vi "VFH, PID Test.vi"() -> ()   [LabVIEW 2016]
uses:
  <vilib>/Platform/TimedLoop/XDataNode/timing_clust.ctl
  <vilib>/Platform/TimedLoop/XDataNode/nitl_modes.ctl
  <vilib>/Platform/TimedLoop/XDataNode/wakeup.ctl
  <vilib>/Utility/AngleManip/Degrees to Radians (Scalar DBL).vi
  <vilib>/addons/control/pid/pid.llb/PID (DBL).vi
  <vilib>/addons/control/pid/pid.llb/PID Lead-Lag (DBL).vi
  <vilib>/Platform/TimedLoop/XDataNode/XDataNode.xnode
  <vilib>/express/express arith-compare/Formula/XNode/ExpressFormulaBlockNode.xnode
  <vilib>/Platform/TimedLoop/XDataNode/XDNodeRunTimeDep.lvlib
  <vilib>/addons/control/pid/NI_PID_pid.lvlib
  <vilib>/Utility/AngleManip/NI_AngleManipulation.lvlib
panel:
  in  "VFH ON/OFF":dbl
  out "Lidar_array":dbl[][](array[numeric])
  out "Encoder Speed_Filtered":dbl format="%#.8g"
  out "IMU Yaw_Filtered":dbl format="%#.8g"
  in  "Q":dbl[][](array[numeric])=[[0.001, 0.0], [0.0, 0.001]]
  in  "R":dbl[][](array[numeric])=[[1e-05, 0.0], [0.0, 1e-05]]
  out "Checksum":bool
  out "Valid":bool
  out "Speed_EKF":dbl
  out "GPS_Speed":dbl
  out "GPS_Heading angle":dbl
  out "Heading_EKF":dbl
  out "GPS_Longitude":dbl
  out "GPS_Latitude":dbl
  out "x_EKF":dbl
  out "y_EKF":dbl
  out "결과":dbl
  out "입력된 속도(protocol)":dbl
  out "Encoder Speed Filtered (m/s)":dbl
  in  "Platform_SPEED(테스트용)":u16
  in  "Lidar shift (m)":dbl=0.48
  in  "Vision shift (m)":dbl=0.87
  out "LIDAR & VISION DATA":cluster{dbl[], dbl[]}(graph)
  in  "Target angle":dbl
  out "Outer Threshold":dbl
  in  "Inner Threshold":dbl=1.5 format="%#_13g"
  in  "거리값 2":dbl
  out "현재 방향각":dbl
  out "Inner Threshold":dbl
  out "입력된 속도 (protocol)":u16
  in  "min speed (protocol)":dbl=35.0 format="%#_13g"
  in  "Global Stop":bool
  in  "Outer Threshold":dbl=0.68
  out "VFH error":bool
  out "PID 입력 브레이크":dbl
  in  "PID gains":T1={"proportional gain (Kc)"=1.0, "integral time (Ti, min)"=0.01, "derivative time (Td, min)"=0.0} caption="PID 게인" {"derivative time (Td, min)" format="%#.6g"; "integral time (Ti, min)" format="%#.6g"; "proportional gain (Kc)" format="%#.6g"}
  out "PV Setpoint Output":cluster{"initial PV":dbl, "setpoint":dbl}(graph)={"initial PV"=0.18693112703744846, "setpoint"=0.0}
  in  "PID 제동거리":dbl=0.5 format="%#_13g"
  in  "max speed (protocol)":dbl=50.0 format="%#_13g"
  in  "obstacle clearance distance":dbl=0.68
  out "mask":bool[](array[boolean])
  out "histogram":dbl[](array[numeric])
  out "Distance":dbl[](array[numeric])
  out "Angle":dbl[](array[numeric])
  in  "출력 클러스터 2":T2
  in  "탭 컨트롤":T3(tab)
  out "Vision Lane":dbl[][](array[numeric])
  out "Lidar 오브젝트화":dbl[][](array[numeric])
  out "Platform Data":i64[](array[numeric])
  out "IMU_Roll":dbl
  out "IMU_Pitch":dbl
  out "IMU_Acceleration":dbl
  out "Total Distance":dbl
  out "Encoder Speed":dbl
  out "IMU_Yaw":dbl
  out "ALIVE":u16
  in  "GEAR":u16(ring) items=["Forward Drive", "Neutral", "Backward Drive"]
  in  "A or M":bool=TRUE
  in  "Platform_E-STOP":bool
  in  "Lidar 오브젝트화 제한 거리(mm)":dbl=200.0
  in  "Lidar 필터 최대거리 (mm)":dbl=25000.0
  in  "Lidar 필터 최소거리 (mm)":dbl=50.0
  in  "GPS port num":refnum<visa-resource-name>="COM9"
  in  "IMU port num":refnum<visa-resource-name>="COM4"
  in  "LIDAR Address":string="192.168.0.204"
  in  "LIDAR port num":u16=2111
  in  "Platform port num":refnum<visa-resource-name>="COM6"
  out "End Loop":bool=TRUE
  # "GPS Data"
  # "IMU, Encoder Data"
  # "KF Data"
  # "EKF Data"
  # "VISION Lane"
  # "LIDAR Obstacle"
  # "Platform Data"
  # "Port Setting"
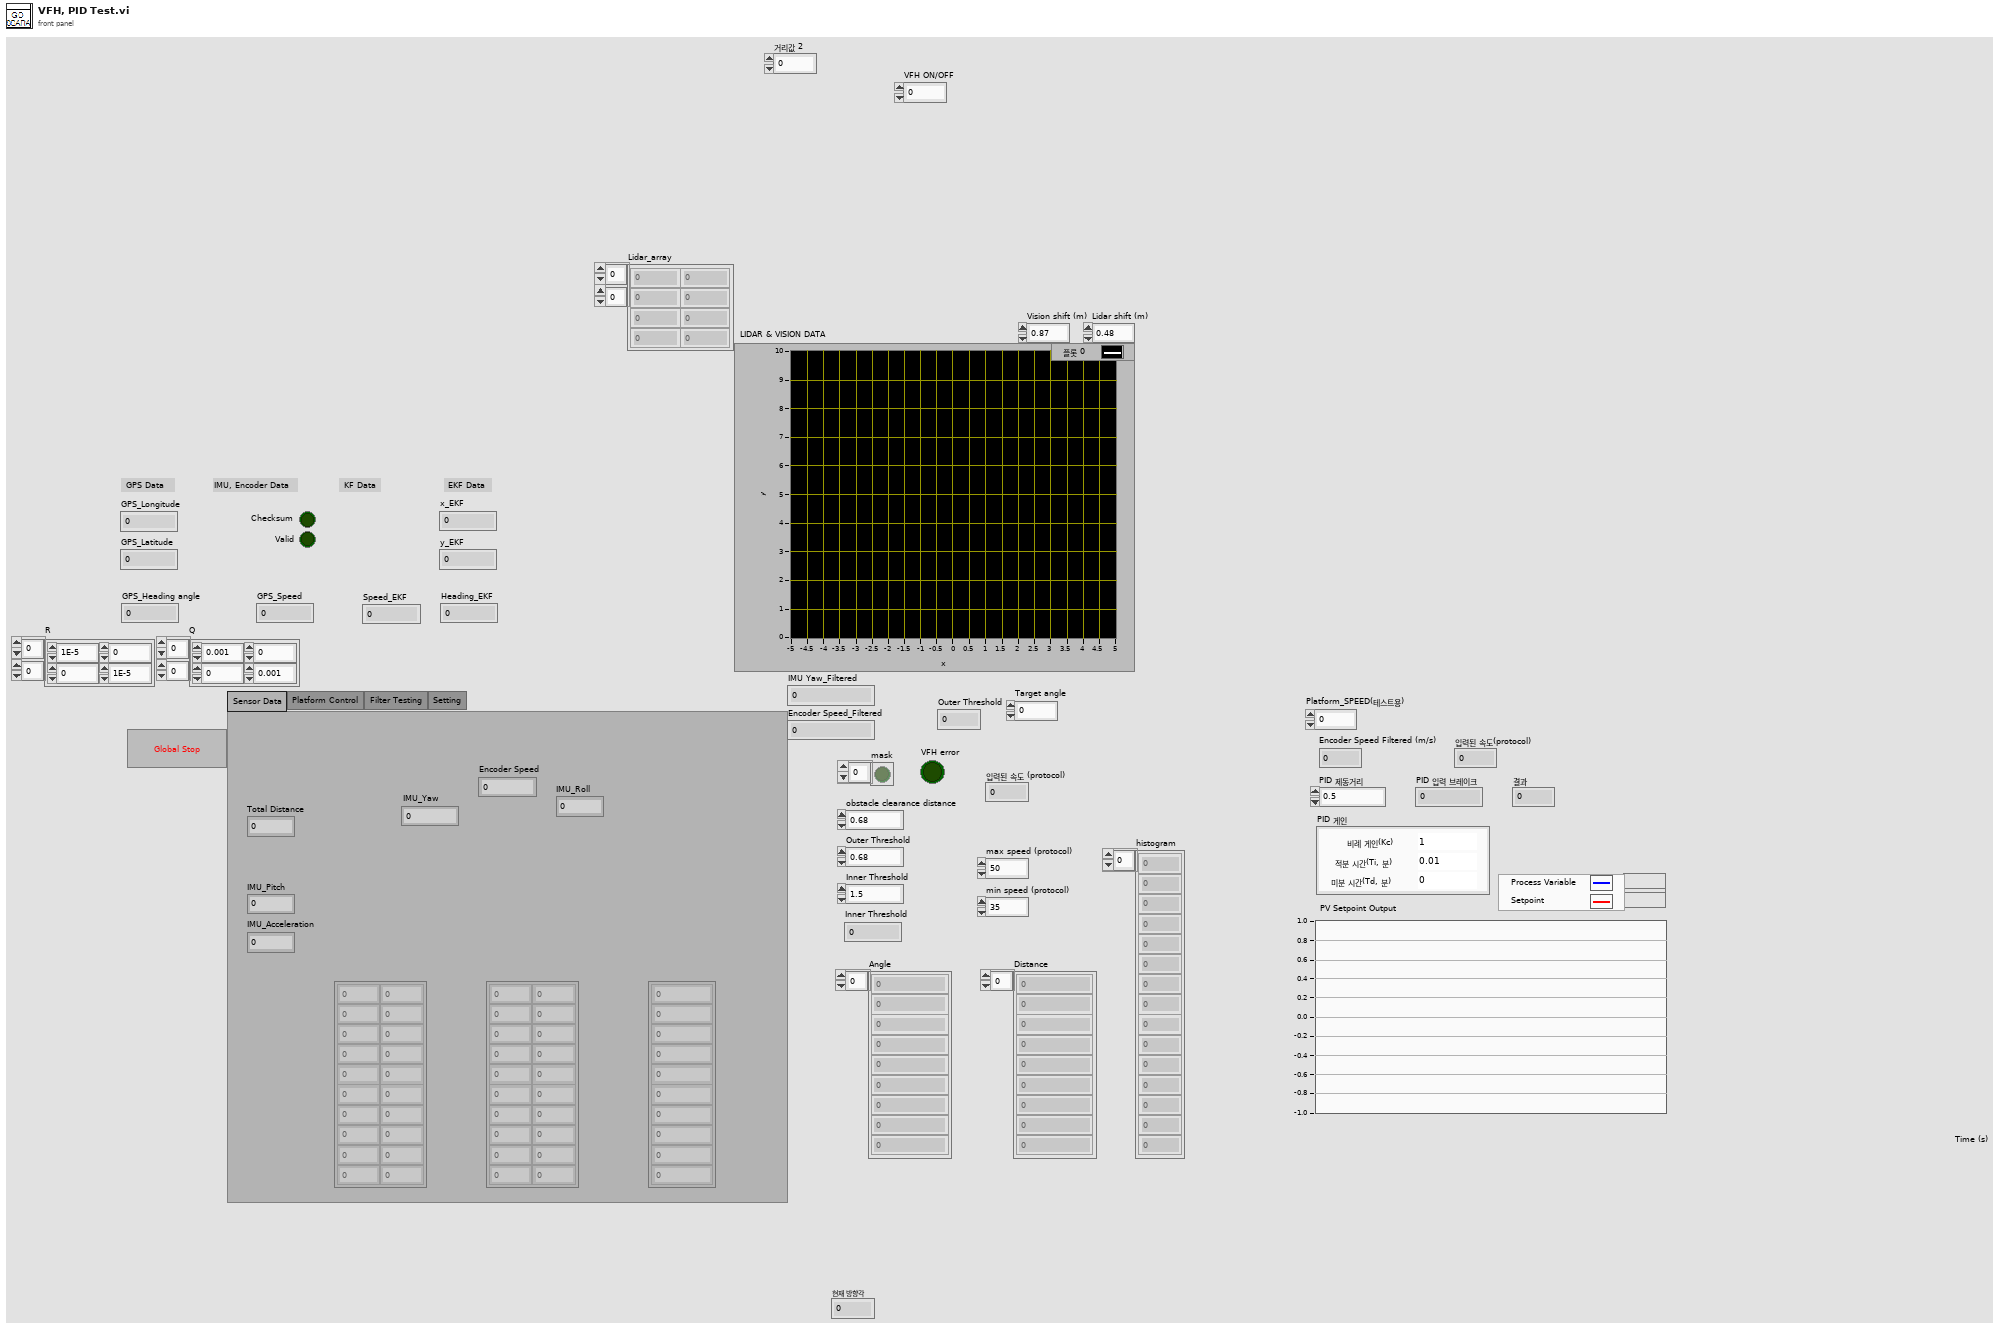
[diagram p1: front panel]
types:
  T1 = cluster{"proportional gain (Kc)":dbl, "integral time (Ti, min)":dbl, "derivative time (Td, min)":dbl}
  T2 = cluster{"Inner Thershold":dbl, "Outer Thershold":dbl}
  T3 = enum32{"Sensor Data", "Platform Control", "Filter Testing", "Setting"}
  T4 = typedef "XDNodeRunTimeDep.lvlib/timing_clust.ctl" = cluster{"Expected End [f-1]":u64, "Actual End [f-1]":u64, "Finished Late? [f-1]":bool, "Expected End [i-1]":u64, "Actual End [i-1]":u64, "Finished Late? [i-1]":bool, "Expected Start [i]":u64, "Actual Start [i]":u64, "Expected Start [f]":u64, "Actual Start [f]":u64, "Source Name":string, "Structure Name":string, "Period":i64, "Deadline":i64, "Offset":i64, "Start":i64, "Priority":i32, "Timeout":i32, "Mode":T5, "Wakeup Reason":T6, "Error":errorcluster, "Source Type":string, "Secondary Source Type":string, "Global End Time":u64, "Global Start Time":u64, "Frame Duration":u64, "Iteration Duration":u64, "Assigned CPU":i32, "I/O Scan Engine Mode":u32}
  T5 = typedef "XDNodeRunTimeDep.lvlib/nitl_modes.ctl" = enum32{"No Change", "Process missed periods, maintain original phase", "Discard missed periods, maintain original phase", "Process missed periods, ignore original phase", "Discard missed periods, ignore original phase"}
  T6 = typedef "XDNodeRunTimeDep.lvlib/wakeup.ctl" = enum32{"Normal", "Aborted", "Asynchronous wakeup", "Timing source error", "Timed loop error", "Timeout"}
  T7 = typedef "2차원배열 공유변수.ctl" = dbl[][]
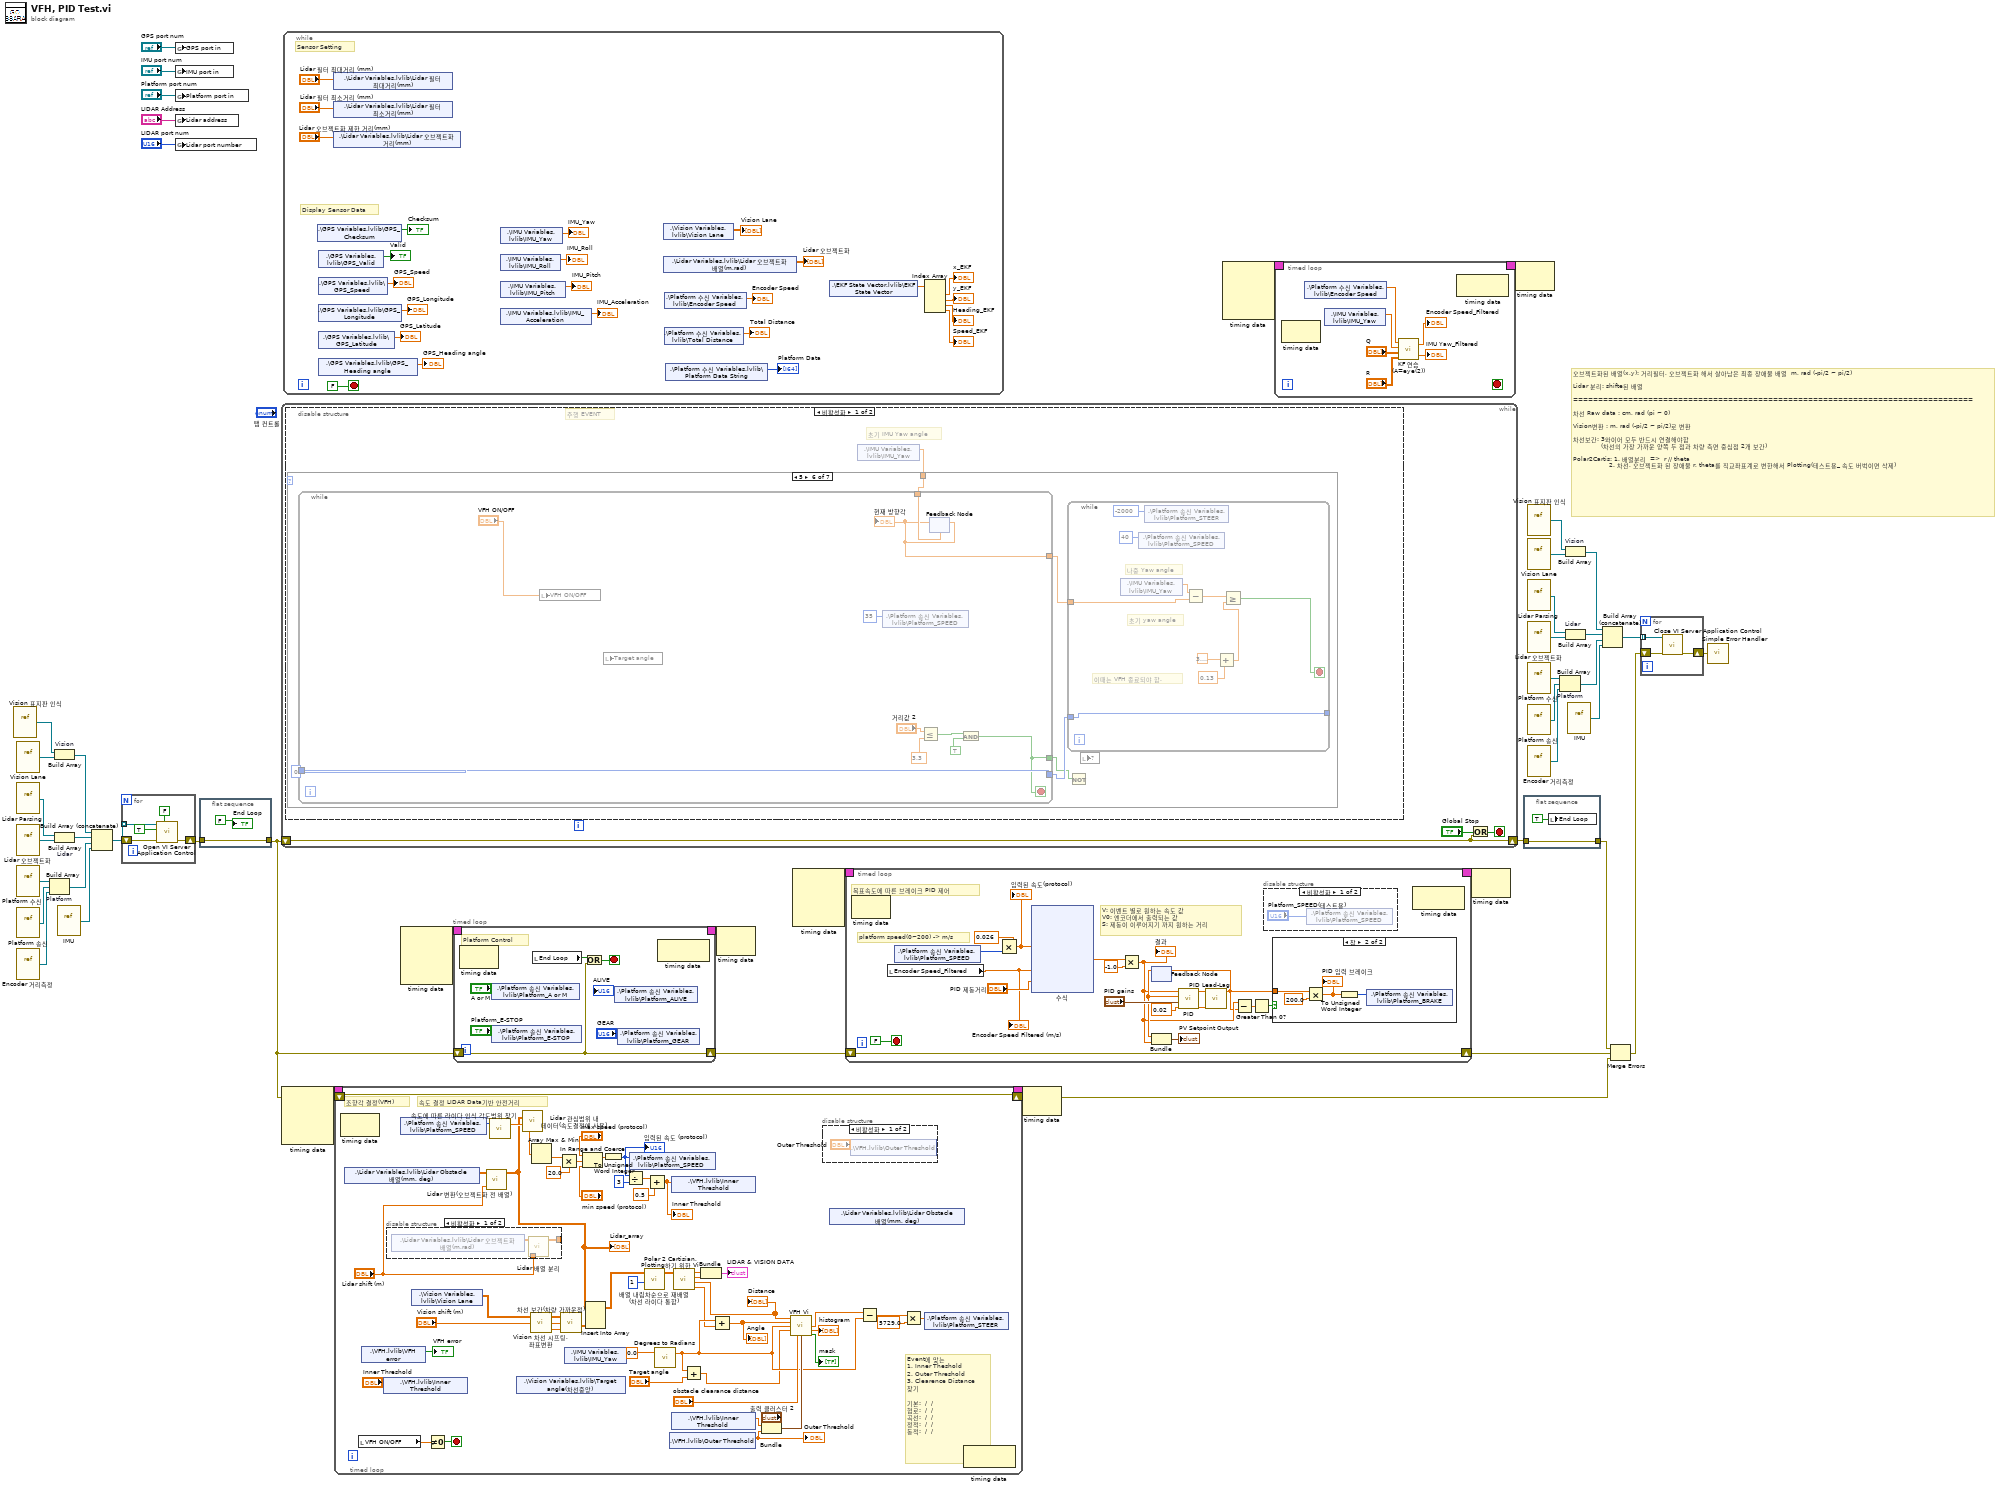
[diagram p0: block diagram]
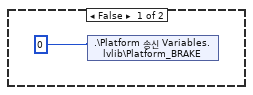
[diagram p5: hidden frame]
diagram:
  # "오브젝트화된 배열(x,y): 거리필터, 오브젝트화 해서 살아남은 최종 장애물 배열  m, rad (-pi/2 ~ pi/2)\n\nLidar 분리: shifte된 배열\n\n================================================================================\n\n차선 Raw data : cm, rad (pi ~ 0) \n\nVision변환 : m, rad (-pi/2 ~ pi/2)로 변환\n\n차선보간: 3와이어 모두 반드시 연결해야함\n              (차선의 가장 가까운 양쪽 두 점과 차량 측면 중심점 2개 보간)\n\nPolar2Cartis: 1. 배열분리  =>  r // theta\n                  2. 차선, 오브젝트화 된 장애물 r, theta를 직교좌표계로 변한해서 Plotting(테스트용_ 속도 버벅이면 삭제)"
  n1 = vi-ref "Vision 표지판 인식.vi"() -> (w1:refnum<vi>)
  n2 = vi-ref "Vision Lane.vi"() -> (w17:refnum<vi>)
  n3 = vi-ref "Lidar Parsing.vi"() -> (w22:refnum<vi>)
  n4 = vi-ref "Lidar 오브젝트화.vi"() -> (w21:refnum<vi>)
  n5 = vi-ref "Platform 수신.vi"() -> (w38:refnum<vi>)
  n6 = vi-ref "Platform 송신.vi"() -> (w37:refnum<vi>)
  n7 = vi-ref "Encoder 거리측정.vi"() -> (w36:refnum<vi>)
  n8 = Build Array "Platform"(w38, w37, w36) -> (w34:refnum<vi>[])
  n9 = Build Array "Vision"(w1, w17) -> (w16:refnum<vi>[])
  n10 = Build Array "Lidar"(w22, w21) -> (w20:refnum<vi>[])
  n11 = vi-ref "IMU.vi"() -> (w35:refnum<vi>)
  n12 = Build Array (concatenate)(w16, w20, w34, w35) -> (w39:refnum<vi>[])
  n13 = for {
    tunnel: w39 -> [w51] mode=indexing
    shift-right: [w48] -> w43
    shift-left: _ -> [w47]
    n14 = call "Open VI Server Application Control.vi"("open front panel (F)"=FALSE ("Open Front Panel"), "error in (no error)"=w47, "run VI (F)"=TRUE ("Run VI"), "VI refnum"=w51) -> ("error out"=w48:errorcluster)  [unwired: 7 in]
  }
  n15 = global write "[GV]_GPS Port NUM.vi" "GPS port in"("GPS port num") -> ()
  n16 = global write "[GV]_IMU Port NUM.vi" "IMU port in"("IMU port num") -> ()
  n17 = global write "[GV]_PLATFORM Port NUM.vi" "Platform port in"("Platform port num") -> ()
  n18 = global write "[GV]_LIDAR Ethernet Address.vi" "Lidar address"("LIDAR Address") -> ()
  n19 = global write "[GV]_LIDAR Port NUM.vi" "Lidar port number"("LIDAR port num") -> ()
  n20 = flat-sequence {
    tunnel: w43 -> [w52]
    tunnel: [w52] -> w6
    frame #0 {
      "End Loop" <- FALSE ("Halt TL")
    }
  }
  n21 = while {
    shift-right: [w55] -> w42
    shift-left: w6 -> [w55]
    stop <- w56 stop-if-true
    n22 = disable-structure shown="비활성화" {
      frame Disabled {
        # "초기 IMU Yaw angle"
        # "주행 EVENT"
        n23 = shared-variable ".\\IMU Variables.lvlib\\IMU_Yaw"() -> (w57:dbl)  [unwired: 1 in, 1 out]
        n24 = case shown="5" {
          selector: _ -> [_ _ _ _ _ _ _]
          tunnel: w57 -> [_ _ _ _ _ w59 _]
          frame 0, Default {
          }
          frame 1 {
          }
          frame 2 {
          }
          frame 3 {
          }
          frame 4 {
          }
          frame 5 {
            n25 = while {
              tunnel: 0 -> [w68]
              tunnel: [w68] -> w60
              tunnel: w59 -> [w67]
              tunnel: [w66] -> w61
              tunnel: [w65] -> w58
              stop <- w65 stop-if-true
              n26 = local write "VFH ON/OFF"("VFH ON/OFF") -> ()
              n27 = local read "Target angle"() -> ()  [unwired: 1 in]
              n28 = shared-variable ".\\Platform 송신 Variables.lvlib\\Platform_SPEED"(u16 35 ("Platform_SPEED")) -> ()  [unwired: 1 in, 1 out]
              n29 = Less Or Equal?(x="거리값 2", y=3.3) -> (x <= y?=w71:bool)
              n30 = feedback #1(w67) -> (w66:dbl)
              "현재 방향각" <- w66
              n31 = feedback-in #1(w66) -> ()
              n32 = And(x=w71, y=TRUE) -> (x .and. y?=w65:bool)
            }
            n33 = while {
              tunnel: w60 -> [w79]
              tunnel: [w79] -> _
              tunnel: w61 -> [w73]
              stop <- w74 stop-if-true
              # "이때는 VFH 종료되야 함."
              # "초기 yaw angle"
              # "나중 Yaw angle"
              n34 = shared-variable ".\\IMU Variables.lvlib\\IMU_Yaw"() -> (w80:dbl)  [unwired: 1 in, 1 out]
              n35 = shared-variable ".\\Platform 송신 Variables.lvlib\\Platform_SPEED"(u16 40 ("Platform_SPEED")) -> ()  [unwired: 1 in, 1 out]
              n36 = shared-variable ".\\Platform 송신 Variables.lvlib\\Platform_STEER"(i16 -2000 ("Platform_STEER")) -> ()  [unwired: 1 in, 1 out]
              n37 = Subtract(x=w80, y=w73) -> (x-y=w76:dbl)
              n38 = Add(x=3.141592653589793, y=0.13) -> (x+y=w75:dbl)
              n39 = Greater Or Equal?(x=w76, y=w75) -> (x >= y?=w74:bool)
            }
            n40 = Not(x=w58) -> ()  [unwired: 1 out]
            n41 = local read item#-1() -> ()  [unwired: 1 in]
          }
          frame 6 {
          }
        }
      }
      frame Enabled {
      }
    }
    n42 = Or(x="Global Stop", y=w55) -> (x .or. y?=w56:bool)
  }
  n43 = node-c288() -> (w8:T4)  [unwired: 4 in]
  n44 = while {
    stop <- FALSE stop-if-true
    # "Sensor Setting"
    # "Display Sensor Data"
    n45 = shared-variable ".\\GPS Variables.lvlib\\GPS_Checksum"() -> (→"Checksum":bool)  [unwired: 1 in, 1 out]
    n46 = shared-variable ".\\GPS Variables.lvlib\\GPS_Valid"() -> (→"Valid":bool)  [unwired: 1 in, 1 out]
    n47 = shared-variable ".\\GPS Variables.lvlib\\GPS_Speed"() -> (→"GPS_Speed":dbl)  [unwired: 1 in, 1 out]
    n48 = shared-variable ".\\GPS Variables.lvlib\\GPS_Longitude"() -> (→"GPS_Longitude":dbl)  [unwired: 1 in, 1 out]
    n49 = shared-variable ".\\GPS Variables.lvlib\\GPS_Latitude"() -> (→"GPS_Latitude":dbl)  [unwired: 1 in, 1 out]
    n50 = shared-variable ".\\GPS Variables.lvlib\\GPS_Heading angle"() -> (→"GPS_Heading angle":dbl)  [unwired: 1 in, 1 out]
    n51 = shared-variable ".\\Lidar Variables.lvlib\\Lidar 필터 최대거리(mm)"("Lidar 필터 최대거리 (mm)") -> ()  [unwired: 1 in, 1 out]
    n52 = shared-variable ".\\Lidar Variables.lvlib\\Lidar 필터 최소거리(mm)"("Lidar 필터 최소거리 (mm)") -> ()  [unwired: 1 in, 1 out]
    n53 = shared-variable ".\\Lidar Variables.lvlib\\Lidar 오브젝트화 거리(mm)"("Lidar 오브젝트화 제한 거리(mm)") -> ()  [unwired: 1 in, 1 out]
    n54 = shared-variable ".\\IMU Variables.lvlib\\IMU_Yaw"() -> (→"IMU_Yaw":dbl)  [unwired: 1 in, 1 out]
    n55 = shared-variable ".\\IMU Variables.lvlib\\IMU_Roll"() -> (→"IMU_Roll":dbl)  [unwired: 1 in, 1 out]
    n56 = shared-variable ".\\IMU Variables.lvlib\\IMU_Pitch"() -> (→"IMU_Pitch":dbl)  [unwired: 1 in, 1 out]
    n57 = shared-variable ".\\IMU Variables.lvlib\\IMU_Acceleration"() -> (→"IMU_Acceleration":dbl)  [unwired: 1 in, 1 out]
    n58 = shared-variable ".\\Vision Variables.lvlib\\Vision Lane"() -> (→"Vision Lane":T7)  [unwired: 1 in, 1 out]
    n59 = shared-variable ".\\Lidar Variables.lvlib\\Lidar 오브젝트화 배열(m,rad)"() -> (→"Lidar 오브젝트화":T7)  [unwired: 1 in, 1 out]
    n60 = shared-variable ".\\Platform 수신 Variables.lvlib\\Encoder Speed"() -> (→"Encoder Speed":dbl)  [unwired: 1 in, 1 out]
    n61 = shared-variable ".\\Platform 수신 Variables.lvlib\\Total Distance"() -> (→"Total Distance":dbl)  [unwired: 1 in, 1 out]
    n62 = shared-variable ".\\Platform 수신 Variables.lvlib\\Platform Data String"() -> (→"Platform Data":i64[])  [unwired: 1 in, 1 out]
    n63 = shared-variable ".\\EKF State Vector.lvlib\\EKF State Vector"() -> (w93:dbl[])  [unwired: 1 in, 1 out]
    n64 = Index Array(array=w93) -> (element #1=→"x_EKF":dbl, element #2=→"y_EKF":dbl, element #3=→"Heading_EKF":dbl, element #4=→"Speed_EKF":dbl)  [unwired: 4 in]
  }
  n65 = timed-loop {
    timing: w8 -> [_]
    timing-out: [_] -> w7
    shift-right: [w110] -> w3
    shift-left: w6 -> [w110]
    stop <- w115 stop-if-true
    # "속도 결정 LIDAR Data기반 안전거리"
    # "조향각 결정(VFH)"
    # "Event에 맞는\n1. Inner Theshold\n2. Outer Threshold\n3. Clearence Distance\n찾기\n\n기본:  /  /  \n협로:  /  /\n곡선:  /  /\n정적:  /  /\n동적:  /  /"
    n66 = node-c288() -> ()  [unwired: 1 in, 1 out]
    n67 = shared-variable ".\\Lidar Variables.lvlib\\Lidar Obstacle 배열(mm, deg)"() -> (w108:T7)  [unwired: 1 in, 1 out]
    n68 = local read "VFH ON/OFF"() -> (w116:dbl)
    n69 = shared-variable ".\\VFH.lvlib\\VFH error"() -> (→"VFH error":bool)  [unwired: 1 in, 1 out]
    n70 = shared-variable ".\\VFH.lvlib\\Inner Threshold"("Inner Threshold") -> ()  [unwired: 1 in, 1 out]
    n71 = disable-structure shown="비활성화" {
      disable-tunnel: "Lidar shift (m)" -> [w161 _]
      disable-tunnel: [w159 _] -> _
      frame Disabled {
        n72 = shared-variable ".\\Lidar Variables.lvlib\\Lidar 오브젝트화 배열(m,rad)"() -> (w160:T7)  [unwired: 1 in, 1 out]
        n73 = call "Lidar 배열 분리.vi"("Lidar shift"=w161, "Lidar"=w160) -> ("Lidar_array"=w159:dbl[][])  [unwired: 1 in, 2 out]
      }
      frame Enabled {
      }
    }
    n74 = shared-variable ".\\Platform 송신 Variables.lvlib\\Platform_SPEED"() -> (w114:u16)  [unwired: 1 in, 1 out]
    n75 = shared-variable ".\\Vision Variables.lvlib\\Vision Lane"() -> (w111:T7)  [unwired: 1 in, 1 out]
    n76 = Not Equal To 0?(x=w116) -> (x != 0?=w115:bool)
    n77 = call "Lidar 변환(오브젝트화 전 배열).vi"("shift"="Lidar shift (m)", "Lidar(오브젝트화 전 배열)"=w108) -> ("X"=w109:dbl[][])  [unwired: 1 in, 2 out]
    "Lidar_array" <- w109
    n78 = call "속도에 따른 라이다 인식 각도범위 찾기.vi"("speed(platform)"=w114) -> ("Interested angle"=w113:dbl)  [unwired: 1 in, 1 out]
    n79 = shared-variable ".\\Vision Variables.lvlib\\Target angle(차선중앙)"() -> ()  [unwired: 1 in, 2 out]
    n80 = call "Lidar 관심범위 내 데이터(속도결정에 사용).vi"("filter angle(plus)"=w113, "Lidar 오브젝트화 후 배열"=w109) -> ("r"=w112:dbl[])  [unwired: 1 in, 2 out]
    n81 = call "Vision 차선 시프팅, 좌표변환.vi"("Vision shift (m)"="Vision shift (m)", "VIsion Lane"=w111) -> ("theta"=w117:dbl[], "r"=w118:dbl[], "Vision"=w119:dbl[][])  [unwired: 1 in]
    n82 = Array Max & Min(array=w112) -> (min value=w124:dbl)  [unwired: 3 out]
    n83 = Multiply(x=w124, y=20.0) -> (x*y=w122:dbl)
    n84 = call "차선 보간(차량 가까운점).vi"("Vision Theta"=w117, "Vision Distance"=w118, "Lane"=w119) -> ("Vision"=w121:dbl[][])  [unwired: 2 out]
    n85 = shared-variable ".\\IMU Variables.lvlib\\IMU_Yaw"() -> ()  [unwired: 1 in, 2 out]
    n86 = In Range and Coerce(upper limit="max speed (protocol)", x=w122, lower limit="min speed (protocol)") -> (coerced(x)=w127:dbl)  [unwired: 1 out]
    n87 = Insert Into Array(array=w109, new element=w121) -> (w141:dbl[][])  [unwired: 2 in]
    n88 = To Unsigned Word Integer(number=w127) -> (unsigned 16bit integer=w128:u16)
    "입력된 속도 (protocol)" <- w128
    n89 = Divide(x=w128, y=u16 3) -> (x/y=w130:dbl)
    n90 = shared-variable ".\\Platform 송신 Variables.lvlib\\Platform_SPEED"(w128) -> ()  [unwired: 1 in, 1 out]
    n91 = call "배열 내림차순으로 재배열 (차선 라이다 통합).vi"("내림차순 기준 인덱스"=1, "입력 배열"=w141) -> ("출력 배열"=w136:dbl[][])  [unwired: 9 in]
    n92 = Add(x=w130, y=0.5) -> (x+y=w132:dbl)
    "Inner Threshold" <- w132
    n93 = call-poly <vilib>:"Degrees to Radians.vi"("angle (deg)"=0.0) -> ("angle (rad)"=w145:dbl)  [unwired: 2 in]
    n94 = shared-variable ".\\VFH.lvlib\\Outer Threshold"() -> (w148:dbl)  [unwired: 1 in, 1 out]
    "Outer Threshold" <- w148
    n95 = shared-variable ".\\VFH.lvlib\\Inner Threshold"() -> (w155:dbl)  [unwired: 1 in, 1 out]
    n96 = shared-variable ".\\VFH.lvlib\\Inner Threshold"(w132) -> ()  [unwired: 1 in, 1 out]
    n97 = call "Polar 2 Cartisian, Plotting하기 위한 Vi.vi"("X"=w136) -> ("theta"=w137:dbl[], "r"=w138:dbl[], "y"=w139:dbl[], "x"=w140:dbl[])  [unwired: 3 in]
    "Distance" <- w138
    n98 = Add(x=w145, y="Target angle") -> (x+y=w135:dbl)
    n99 = Bundle("x"=w140, "y"=w139) -> (→"LIDAR & VISION DATA":cluster{"x":dbl[], "y":dbl[]})  [unwired: 1 in]
    n100 = Add(x=w145, y=w137) -> (x+y=w150:dbl[])
    "Angle" <- w150
    n101 = Bundle(cluster="출력 클러스터 2", "Inner Thershold"=w155, "Outer Thershold"=w148) -> (w154:T2)
    n102 = call "VFH Vi.vi"("LIDAR & Vision magn. (m)"=w138, "LIDAR & Vision angle (rad)"=w150, "current heading (rad)"=w145, "target heading (rad)"=w135, "obstacle clearance (m)"="obstacle clearance distance", "thresholds"=w154) -> ("command heading (rad)"=w149:dbl, "histogram out"=→"histogram":dbl[], "mask out"=→"mask":bool[])  [unwired: 7 in]
    n103 = disable-structure shown="비활성화" {
      frame Disabled {
        n104 = shared-variable ".\\VFH.lvlib\\Outer Threshold"("Outer Threshold") -> ()  [unwired: 1 in, 1 out]
      }
      frame Enabled {
      }
    }
    n105 = shared-variable ".\\Lidar Variables.lvlib\\Lidar Obstacle 배열(mm, deg)"() -> ()  [unwired: 1 in, 2 out]
    n106 = Subtract(x=w149, y=w145) -> (x-y=w157:dbl)
    n107 = Multiply(x=w157, y=5729.0) -> (x*y=w147:dbl)
    n108 = shared-variable ".\\Platform 송신 Variables.lvlib\\Platform_STEER"(w147) -> ()  [unwired: 1 in, 1 out]
    n109 = node-c288() -> ()  [unwired: 1 in, 1 out]
  }
  n110 = node-c288() -> (w46:T4)  [unwired: 4 in]
  n111 = timed-loop {
    timing: w46 -> [_]
    timing-out: [_] -> w45
    shift-right: [w170] -> w5
    shift-left: w6 -> [w170]
    stop <- w171 stop-if-true
    # "Platform Control"
    n112 = node-c288() -> ()  [unwired: 1 in, 1 out]
    n113 = shared-variable ".\\Platform 송신 Variables.lvlib\\Platform_A or M"("A or M") -> ()  [unwired: 1 in, 1 out]
    n114 = shared-variable ".\\Platform 송신 Variables.lvlib\\Platform_E-STOP"("Platform_E-STOP") -> ()  [unwired: 1 in, 1 out]
    n115 = local read "End Loop"() -> (w169:bool)
    n116 = Or(x=w169, y=w170) -> (x .or. y?=w171:bool)
    n117 = shared-variable ".\\Platform 송신 Variables.lvlib\\Platform_ALIVE"() -> (→"ALIVE":u16)  [unwired: 1 in, 1 out]
    n118 = shared-variable ".\\Platform 송신 Variables.lvlib\\Platform_GEAR"("GEAR") -> ()  [unwired: 1 in, 1 out]
    n119 = node-c288() -> ()  [unwired: 1 in, 1 out]
  }
  n120 = node-c288(w45) -> ()  [unwired: 1 out]
  n121 = node-c288() -> (w19:T4)  [unwired: 4 in]
  n122 = timed-loop {
    timing: w19 -> [_]
    timing-out: [_] -> w18
    shift-right: [w174] -> w4
    shift-left: w5 -> [w174]
    stop <- FALSE stop-if-true
    # "platform speed(0~200) -> m/s"
    # "목표속도에 따른 브레이크 PID 제어"
    # "V: 이벤트 별로 원하는 속도 값\nV0: 엔코더에서 출력되는 값\nS: 제동이 이루어지기 까지 원하는 거리"
    n123 = node-c288() -> ()  [unwired: 1 in, 1 out]
    n124 = local read "Encoder Speed_Filtered"() -> (w175:dbl)
    "Encoder Speed Filtered (m/s)" <- w175
    n125 = shared-variable ".\\Platform 송신 Variables.lvlib\\Platform_SPEED"() -> (w176:u16)  [unwired: 1 in, 1 out]
    n126 = Multiply(x=0.026, y=w176) -> (x*y=w179:dbl)
    "입력된 속도(protocol)" <- w179
    n127 = xnode "수식"("V"=w179, "V0"=w175, "S"="PID 제동거리") -> ("결과"=w184:dbl)  [unwired: 1 in, 1 out]
    n128 = Multiply(x=w184, y=-1.0) -> (x*y=w182:dbl)
    "결과" <- w182
    n129 = feedback #2() -> (w190:dbl)  [unwired: 1 in]
    n130 = Bundle("output"=w190, w182) -> (→"PV Setpoint Output":cluster{"output":dbl, dbl})  [unwired: 1 in]
    n131 = call-poly <vilib>:"PID.vi"("dt (s)"=0.02, "PID gains"="PID gains", "process variable"=w190, "setpoint"=w182) -> ("dt out (s)"=w188:dbl, "output"=w187:dbl)  [unwired: 6 in]
    n132 = call-poly <vilib>:"PID Lead-Lag.vi"("dt (s)"=w188, "input"=w187) -> ("output"=w181:dbl)  [unwired: 6 in, 1 out]
    n133 = feedback-in #2(w181) -> ()
    n134 = Subtract(x=w182, y=w181) -> (x-y=w180:dbl)
    n135 = Greater Than 0?(x=w180) -> (x > 0?=w183:bool)
    n136 = disable-structure shown="비활성화" {
      frame Disabled {
        n137 = shared-variable ".\\Platform 송신 Variables.lvlib\\Platform_SPEED"("Platform_SPEED(테스트용)") -> ()  [unwired: 1 in, 1 out]
      }
      frame Enabled {
      }
    }
    n138 = case shown="참" w183 {
      tunnel: w181 -> [_ w210]
      frame False {
        n139 = shared-variable ".\\Platform 송신 Variables.lvlib\\Platform_BRAKE"(i16 0 ("brake")) -> ()  [unwired: 1 in, 1 out]
      }
      frame True {
        n140 = Multiply(x=w210, y=200.0) -> (x*y=w208:dbl)
        "PID 입력 브레이크" <- w208
        n141 = To Unsigned Word Integer(number=w208) -> (unsigned 16bit integer=w207:u16)
        n142 = shared-variable ".\\Platform 송신 Variables.lvlib\\Platform_BRAKE"(w207) -> ()  [unwired: 1 in, 1 out]
      }
    }
    n143 = node-c288() -> ()  [unwired: 1 in, 1 out]
  }
  n144 = node-c288(w7) -> ()  [unwired: 1 out]
  n145 = node-c288() -> (w27:T4)  [unwired: 4 in]
  n146 = timed-loop {
    timing: w27 -> [_]
    timing-out: [_] -> w26
    stop <- _ stop-if-true
    n147 = node-c288() -> ()  [unwired: 1 in, 1 out]
    n148 = shared-variable ".\\Platform 수신 Variables.lvlib\\Encoder Speed"() -> (w217:dbl)  [unwired: 1 in, 1 out]
    n149 = shared-variable ".\\IMU Variables.lvlib\\IMU_Yaw"() -> (w218:dbl)  [unwired: 1 in, 1 out]
    n150 = call "KF 연습 (A=eye(2)).vi"("R"="R", "Q"="Q", "Y_input"=w218, "X_input"=w217) -> ("Y_Filtered"=→"IMU Yaw_Filtered":dbl, "X_Filtered"=→"Encoder Speed_Filtered":dbl)
    n151 = node-c288() -> ()  [unwired: 1 in, 1 out]
  }
  n152 = node-c288(w18) -> ()  [unwired: 1 out]
  n153 = node-c288(w26) -> ()  [unwired: 1 out]
  n154 = flat-sequence {
    tunnel: w42 -> [w222]
    tunnel: [w222] -> w41
    frame #0 {
      n155 = local write "End Loop"(TRUE ("End Loop")) -> ()
    }
  }
  n156 = vi-ref "Lidar Parsing.vi"() -> (w25:refnum<vi>)
  n157 = vi-ref "Lidar 오브젝트화.vi"() -> (w24:refnum<vi>)
  n158 = vi-ref "Platform 수신.vi"() -> (w33:refnum<vi>)
  n159 = vi-ref "Platform 송신.vi"() -> (w32:refnum<vi>)
  n160 = vi-ref "Encoder 거리측정.vi"() -> (w31:refnum<vi>)
  n161 = vi-ref "Vision 표지판 인식.vi"() -> (w2:refnum<vi>)
  n162 = vi-ref "Vision Lane.vi"() -> (w15:refnum<vi>)
  n163 = Build Array "Platform"(w33, w32, w31) -> (w29:refnum<vi>[])
  n164 = Build Array "Vision"(w2, w15) -> (w14:refnum<vi>[])
  n165 = Build Array "Lidar"(w25, w24) -> (w23:refnum<vi>[])
  n166 = vi-ref "IMU.vi"() -> (w30:refnum<vi>)
  n167 = Build Array (concatenate)(w14, w23, w29, w30) -> (w28:refnum<vi>[])
  n168 = Merge Errors(w41, w4, w3) -> (w40:errorcluster)
  n169 = for {
    tunnel: w28 -> [w223] mode=indexing
    shift-right: [w225] -> w44
    shift-left: w40 -> [w224]
    n170 = call "Close VI Server Application Control.vi"("error in (no error)"=w224, "VI refnum"=w223) -> ("error out"=w225:errorcluster)  [unwired: 9 in]
  }
  n171 = call <vilib>:"Simple Error Handler.vi"("error in (no error)"=w44) -> ()  [unwired: 4 in, 5 out]
